vi "Ignore Error 56.vi"(8 "error in (no error)":errorcluster) -> (0 "error out":errorcluster)   [LabVIEW 2015, in "niDTS CommLib.lvlib" / "niDTS Comm Telnet.lvclass"]
uses:
  niDTS Comm Telnet.lvclass
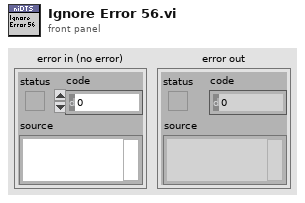
[diagram p1: front panel]
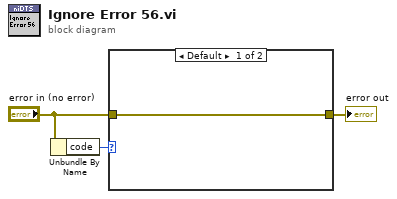
[diagram p0: block diagram]
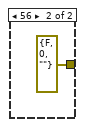
[diagram p2: hidden frame]
diagram:
  n1 = Unbundle By Name("error in (no error)") -> ("code"=w2:i32)
  n2 = case shown="Default" w2 {
    tunnel: "error in (no error)" -> [w4 _]
    tunnel: [w4 errorcluster {"status"=FALSE, "code"=0, "source"=""} ("error in")] -> w1
    frame Default {
    }
    frame 56 {
    }
  }
  "error out" <- w1
